vi "macro_FiniteStateMachine_Template.vi"   [LabVIEW 2019, in "Trajectory_Library.lvlib"]
uses:
  Trajectory_Library.lvlib
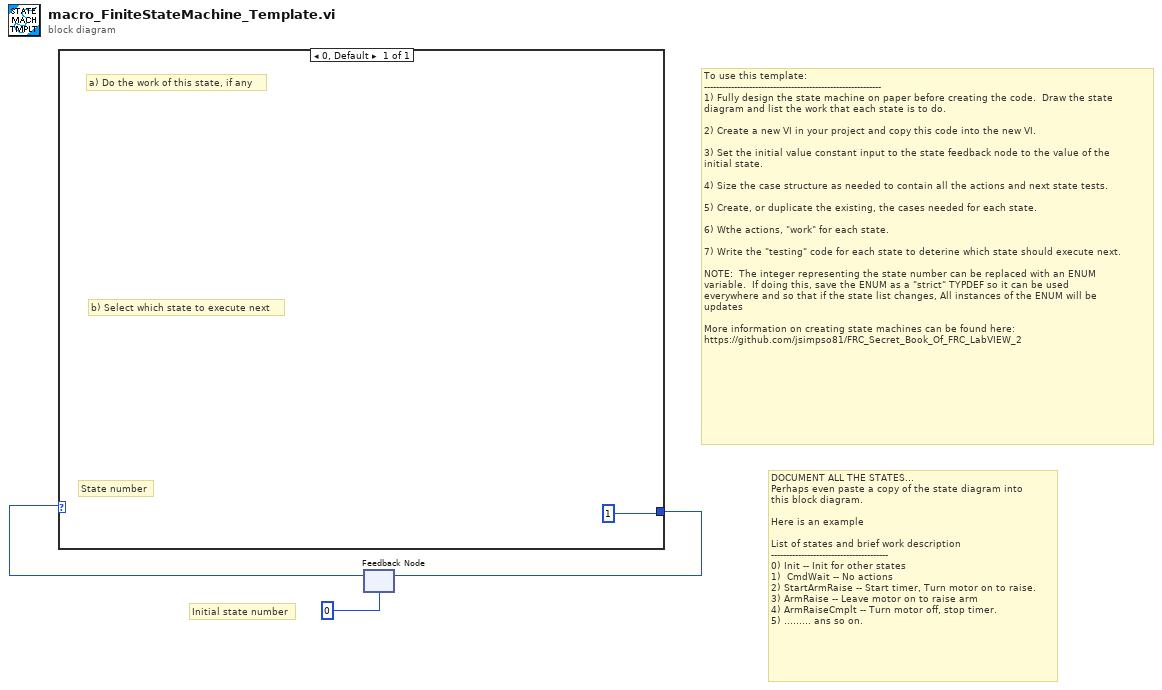
[diagram p0: block diagram]
diagram:
  # "DOCUMENT ALL THE STATES...  \nPerhaps even paste a copy of the state diagram into\nthis block diagram.\n\nHere is an example\n\nList of states and brief work description\n---------------------------------------\n0) Init -- Init for other states\n1)  CmdWait -- No actions\n2) StartArmRaise -- Start timer, Turn motor on to raise.\n3) ArmRaise -- Leave motor on to raise arm\n4) ArmRaiseCmplt -- Turn motor off, stop timer.\n5) ......... ans so on."
  # "Initial state number"
  # "To use this template:\n-----------------------------------------------------------\n1) Fully design the state machine on paper before creating the code.  Draw the state\ndiagram and list the work that each state is to do.\n\n2) Create a new VI in your project and copy this code into the new VI.\n\n3) Set the initial value constant input to the state feedback node to the value of the\ninitial state.\n\n4) Size the case structure as needed to contain all the actions and next state tests.  \n\n5) Create, or duplicate the existing, the cases needed for each state.  \n\n6) Wthe actions, \"work\" for each state.\n\n7) Write the \"testing\" code for each state to deterine which state should execute next.\n\nNOTE:  The integer representing the state number can be replaced with an ENUM \nvariable.  If doing this, save the ENUM as a \"strict\" TYPDEF so it can be used \neverywhere and so that if the state list changes, All instances of the ENUM will be\nupdates\n\nMore information on creating state machines can be found here:\nhttps://github.com/jsimpso81/FRC_Secret_Book_Of_FRC_LabVIEW_2"
  n1 = feedback #1(u32 0) -> (w2:u32)
  n2 = case shown="0, Default" w2 {
    tunnel: [u32 1] -> w1
    frame 0, Default {
      # "State number"
      # "b) Select which state to execute next"
      # "a) Do the work of this state, if any"
    }
  }
  n3 = feedback-in #1(w1) -> ()
